vi "Control_Twin_SourceQ.vi"(0 "Control":T2(ring), 1 "Source2 Flowrate l/min":dbl, 2 "Mode":T1) -> ()   [LabVIEW 2020]
uses:
  ADAM Client/Sub VIs/ADAM Controls/Update_scan_value.ctl
  Controls/User_Specific_mode.ctl
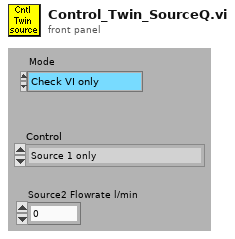
[diagram p1: front panel]
types:
  T1 = typedef "User_Specific_mode.ctl" = enum16{"Check VI only", "Run VI"}
  T2 = enum16{"Source 1 only", "Source 2 only", "Both Sources"}
  T3 = typedef "Update_scan_value.ctl" = cluster{"Channel Name":string, "New Value":dbl}
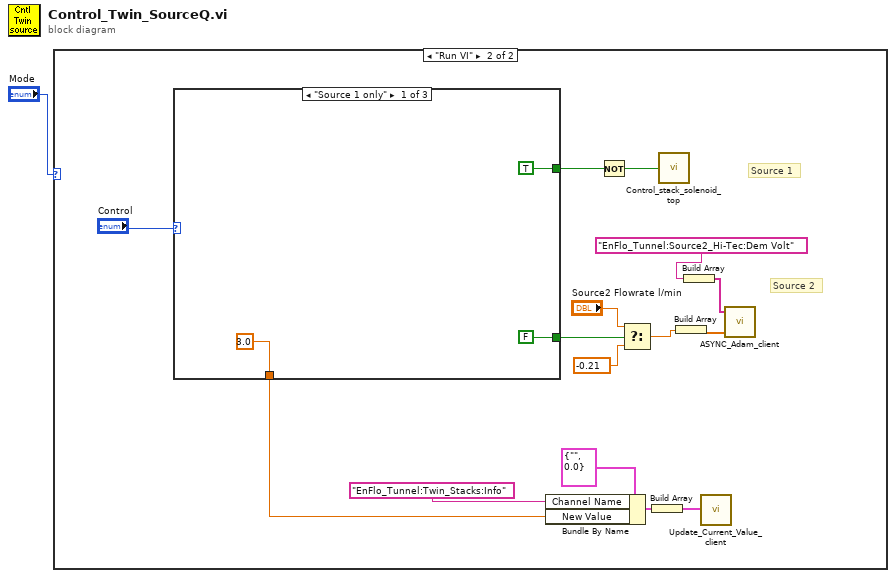
[diagram p0: block diagram]
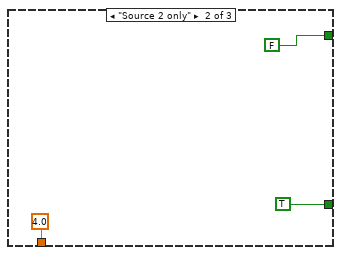
[diagram p3: hidden frame]
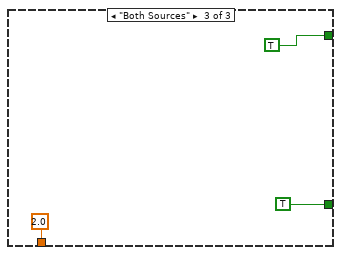
[diagram p4: hidden frame]
diagram:
  n1 = case shown="\"Run VI\"" "Mode" {
    frame "Check VI only" {
    }
    frame "Run VI" {
      # "Source 2"
      # "Source 1"
      n2 = case shown="\"Source 1 only\"" "Control" {
        tunnel: [TRUE FALSE TRUE] -> w10
        tunnel: [FALSE TRUE TRUE] -> w9
        tunnel: [3.0 4.0 2.0] -> w4
        frame "Source 1 only" {
        }
        frame "Source 2 only" {
        }
        frame "Both Sources" {
        }
      }
      n3 = Bundle By Name(cluster=T3 {"Channel Name"="", "New Value"=0.0} ("Update Scan Value Cluster"), "Channel Name"="EnFlo_Tunnel:Twin_Stacks:Info", "New Value"=w4) -> (w7:T3)
      n4 = Not(x=w10) -> (.not. x?=w3:bool)
      n5 = Select(t="Source2 Flowrate l/min", s=w9, f=-0.21) -> (s? t:f=w13:dbl)
      n6 = Build Array(w7) -> (w6:T3[])
      n7 = call "Control_stack_solenoid_top.vi"("Valve On?"=w3) -> ()  [unwired: 2 out]
      n8 = Build Array(w13) -> (w12:dbl[])
      n9 = Build Array("EnFlo_Tunnel:Source2_Hi-Tec:Dem Volt") -> (w15:string[])
      n10 = call "Update_Current_Value_client.vi"("Update array in"=w6) -> ()  [unwired: 1 in]
      n11 = call "ASYNC_Adam_client.vi"("Values"=w12, "Channel Names"=w15) -> ()  [unwired: 1 in, 2 out]
    }
  }
